vi "New line trigger.vi"(7 "MC":bool, 8 "New line trigger enabled":bool, 9 "aod_fill_active in":bool, 10 "refscan_next":bool, 11 "AQ STATE":T1=enum."Wait N after Trigger") -> (3 "aod_fill_active":bool)   [LabVIEW 2020]
uses:
  FPGA Typedefs/Image State.ctl
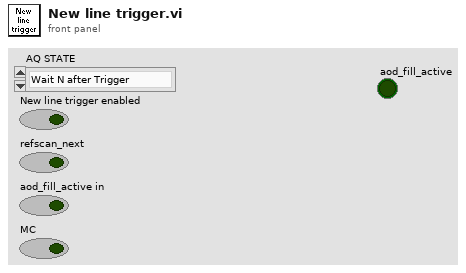
[diagram p1: front panel]
types:
  T1 = typedef "Image State.ctl" = enum16{"Start Up", "Wait for Trigger", "Wait N after Trigger", "DAQ Pointing", "DAQ Scan", "Reference Scan", "Pointing AOL Fill", "Scan AOL FILL", "Reference AOL Fill"}
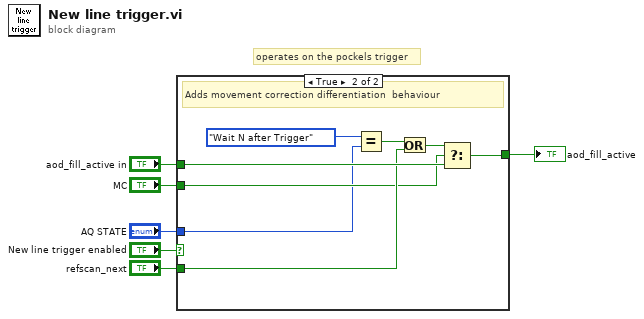
[diagram p0: block diagram]
diagram:
  # "operates on the pockels trigger"
  n1 = case shown="True" "New line trigger enabled" {
    tunnel: "aod_fill_active in" -> [w7 w15]
    tunnel: [w7 w14] -> w3
    tunnel: "AQ STATE" -> [_ w9]
    tunnel: "refscan_next" -> [_ w12]
    tunnel: "MC" -> [_ w10]
    frame False {
      # "Default"
    }
    frame True {
      # "Adds movement correction differentiation  behaviour"
      n2 = Equal?(x=Image_State."Wait N after Trigger" ("Enum"), y=w9) -> (x = y?=w13:bool)
      n3 = Or(x=w13, y=w12) -> (x .or. y?=w11:bool)
      n4 = Select(t=w11, s=w10, f=w15) -> (s? t:f=w14:bool)
    }
  }
  "aod_fill_active" <- w3
